vi "Connect.vi"(8 "error in (no error)":errorcluster, 11 "Module ID":i32=-1) -> (0 "error out":errorcluster)   [LabVIEW 2014, in "GenNet-Client.lvlib"]
doc: "Open the TCP/IP connection to the listening module\n_____\nCreated using Delacor QMH Event Scripter 4.0.0.65."
uses:
  GenNet-Client.lvlib
  Connect Argument--cluster.ctl
  Connect (Reply Payload)--cluster.ctl
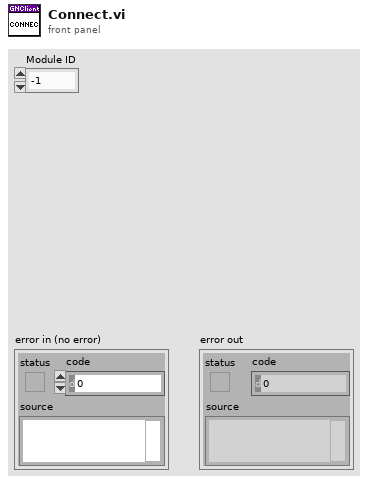
[diagram p1: front panel]
types:
  T1 = typedef "GenNet-Client.lvlib/Connect Argument--cluster.ctl" = cluster{"Module ID":i32, "Wait Notifier":refnum<notifier>}
  T2 = typedef "GenNet-Client.lvlib/Request Events--cluster.ctl" = cluster{"Stop Module":refnum<user-event>, "Show Panel":refnum<user-event>, "Hide Panel":refnum<user-event>, "Show Diagram":refnum<user-event>, "Get Module Execution Status":refnum<user-event>, "Send via Network":refnum<user-event>, "Connect":refnum<user-event>, "Listen for Network Broadcasts":refnum<user-event>}
  T3 = typedef "GenNet-Client.lvlib/Connect (Reply Payload)--cluster.ctl" = cluster{"error":errorcluster}
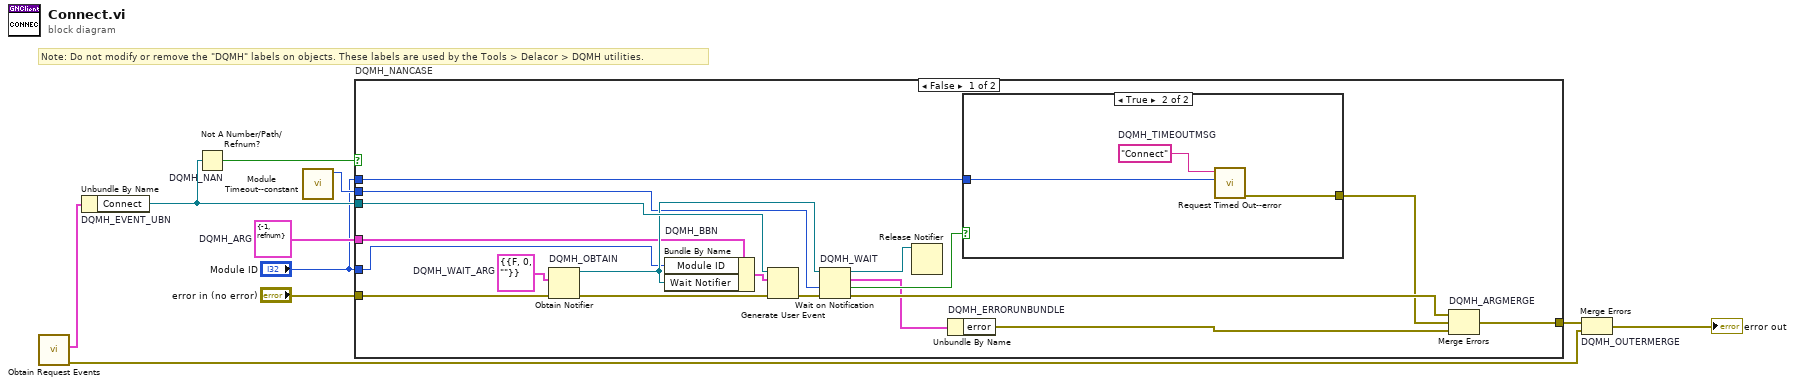
[diagram p0: block diagram]
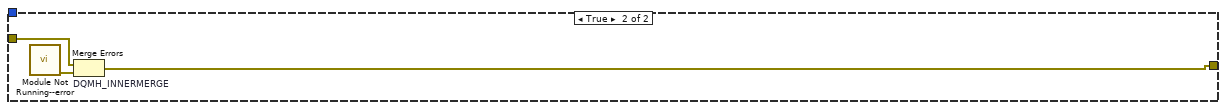
[diagram p3: hidden frame]
diagram:
  w5 = T1 {"Module ID"=-1, "Wait Notifier"=refnum}  # DQMH_ARG
  # "Note: Do not modify or remove the \"DQMH\" labels on objects. These labels are used by the Tools > Delacor > DQMH utilities."
  n1 = call "Obtain Request Events.vi"() -> ("error out"=w2:errorcluster, "GenNet-Client Request Events"=w1:T2)  [unwired: 10 in]
  n2 = Unbundle By Name "DQMH_EVENT_UBN"(w1) -> ("Connect"=w8:refnum<user-event>)
  n3 = Not A Number/Path/Refnum? "DQMH_NAN"(number/path/refnum=w8) -> (NaN/Path/Refnum?=w7:bool)
  n4 = call "Module Timeout--constant.vi"() -> ("Module Timeout"=w4:i32)  [unwired: 11 in]
  n5 = case "DQMH_NANCASE" shown="False" w7 {
    tunnel: "error in (no error)" -> [w28 w34]
    tunnel: w8 -> [w26 _]
    tunnel: [w19 w33] -> w6
    tunnel: w5 -> [w15 _]
    tunnel: "Module ID" -> [w14 _]
    tunnel: w4 -> [w13 _]
    tunnel: "Module ID" -> [w12 _]
    frame False {
      w24 = T3 {"error"={"status"=FALSE, "code"=0, "source"=""}}  # DQMH_WAIT_ARG
      n6 = Obtain Notifier "DQMH_OBTAIN"(notification data type=w24, error in (no error)=w28) -> (notifier out=w22:refnum<notifier>, error out=w25:errorcluster)  [unwired: 2 in, 1 out]
      n7 = Bundle By Name "DQMH_BBN"(cluster=w15, "Module ID"=w14, "Wait Notifier"=w22) -> (w16:T1)
      n8 = Generate User Event(user event=w26, event data cluster=w16, error in=w25) -> (error out=w27:errorcluster)  [unwired: 1 in, 1 out]
      n9 = Wait on Notification "DQMH_WAIT"(notifier=w22, timeout in ms (-1)=w13, error in (no error)=w27) -> (notifier out=w21:refnum<notifier>, notification=w17:T3, timed out?=w20:bool, error out=w23:errorcluster)  [unwired: 1 in]
      n10 = Release Notifier(notifier=w21) -> ()  [unwired: 2 in, 3 out]
      n11 = Unbundle By Name "DQMH_ERRORUNBUNDLE"(w17) -> ("error"=w18:errorcluster)
      n12 = case shown="True" w20 {
        tunnel: w12 -> [_ w31]
        tunnel: [_ w29] -> w11
        frame False {
        }
        frame True {
          w30 = "Connect"  # DQMH_TIMEOUTMSG
          n13 = call "Request Timed Out--error.vi"("Module ID"=w31, "Request"=w30) -> ("error out"=w29:errorcluster)  [unwired: 9 in]
        }
      }
      n14 = Merge Errors "DQMH_ARGMERGE"(w23, w11, w18) -> (w19:errorcluster)
    }
    frame True {
      n15 = call "Module Not Running--error.vi"() -> ("error out"=w32:errorcluster)  [unwired: 11 in]
      n16 = Merge Errors "DQMH_INNERMERGE"(w34, w32) -> (w33:errorcluster)
    }
  }
  n17 = Merge Errors "DQMH_OUTERMERGE"(w6, w2) -> (→"error out":errorcluster)
